vi "ke2002_config_4wR.vi"(7 "range value (ohms)":dbl, 8 "error in":errorcluster, 11 "VISA in":refnum<visa-resource-name>) -> (0 "error out":errorcluster, 3 "VISA out":refnum<visa-resource-name>)   [LabVIEW 2020]
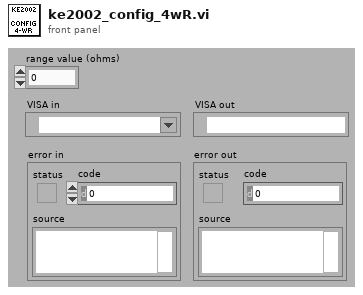
[diagram p1: front panel]
types:
  T1 = cluster{"error":bool, "code":i32, "source":string}
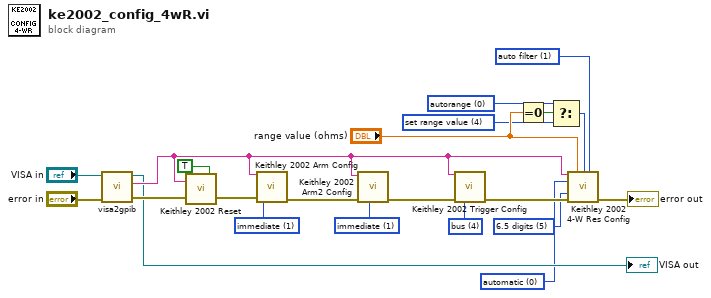
[diagram p0: block diagram]
diagram:
  w1 = u16 0 items=["autorange", "autorange once", "set min range", "set max range", "set range value"] ("range (auto:0)")
  w6 = u16 0 items=["automatic", "automatic once", "set to minimum", "set to maximum", "set aperature value", "set NPLC value"] ("integration time (0:auto)")
  w13 = u16 1 items=["off", "auto filter", "auto filter once", "moving filter", "repeating filter"] ("digital filter (off:0)")
  w14 = u16 5 items=["auto resolution", "auto resolution once", "3.5 digits", "4.5 digits", "5.5 digits", "6.5 digits", "7.5 digits", "8.5 digits"] ("resolution (4.5 digits:3)")
  w2 = u16 4 items=["autorange", "autorange once", "set min range", "set max range", "set range value"] ("range (auto:0)")
  w16 = u16 4 items=["hold", "immediate", "timer", "manual", "bus", "trigger link", "external"] ("source (imm:1)")
  w18 = u16 1 items=["hold", "immediate", "timer", "manual", "bus", "trigger link", "external"] ("source (imm:1)")
  w19 = u16 1 items=["hold", "immediate", "manual", "bus", "trigger link", "external", "Real-Time Clock"] ("source (imm:1)")
  n1 = call "visa2gpib.vi"("error in"="error in", "VISA in"="VISA in") -> ("error out"=w12:errorcluster, "combined address"=w10:string, "VISA out"=→"VISA out":refnum<visa-resource-name>)  [unwired: 7 in]
  n2 = call "Keithley 2002 Reset.vi"("reset/preset"=TRUE, "error in"=w12, "GPIB address"=w10) -> ("error out"=w11:T1)
  n3 = call "Keithley 2002 Arm Config.vi"("GPIB address"=w10, "source (imm:1)"=w19, "error in"=w11) -> ("error out"=w20:T1)  [unwired: 12 in]
  n4 = call "Keithley 2002 Arm2 Config.vi"("source (imm:1)"=w18, "error in"=w20, "GPIB address"=w10) -> ("error out"=w17:T1)  [unwired: 8 in]
  n5 = call "Keithley 2002 Trigger Config.vi"("GPIB address"=w10, "error in"=w17, "source (imm:1)"=w16) -> ("error out"=w15:T1)  [unwired: 12 in]
  n6 = Equal To 0?(x="range value (ohms)") -> (x = 0?=w4:bool)
  n7 = Select(t=w1, s=w4, f=w2) -> (s? t:f=w5:u16)
  n8 = call "Keithley 2002 4-W Res Config.vi"("GPIB address"=w10, "range value (ohms)"="range value (ohms)", "range (auto:0)"=w5, "digital filter (off:0)"=w13, "integration time (0:auto)"=w6, "resolution (4.5 digits:3)"=w14, "error in"=w15) -> ("error out"=→"error out":T1)  [unwired: 8 in]
